vi "Run.vi"(8 "error in (no error)":errorcluster, 11 "Channel Rep in":refnum<class "Channel Rep.lvclass">) -> (0 "error out":errorcluster, 3 "Channel Rep out":refnum<class "Channel Rep.lvclass">)   [LabVIEW 2018, in "Channel Rep.lvclass"]
uses:
  Channel Rep.lvclass
  State Machine/State Machine.lvclass
  Socket2/Socket2/Socket2.lvclass
  RxTx/RxTx.lvclass
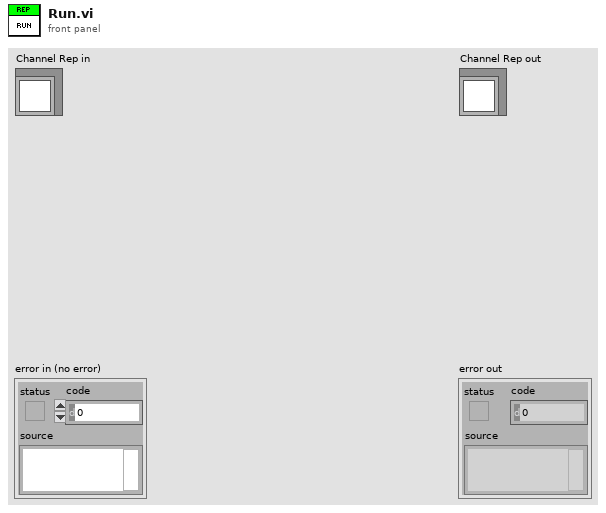
[diagram p1: front panel]
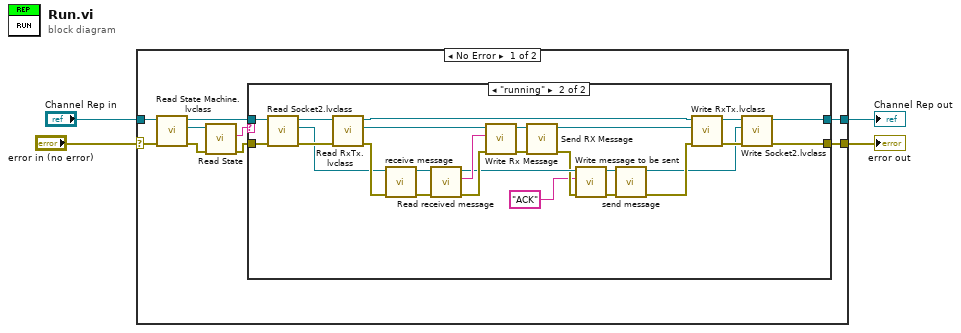
[diagram p0: block diagram]
diagram:
  n1 = case shown="No Error" "error in (no error)" {
    selector: "error in (no error)" -> [w12 w42]
    tunnel: "Channel Rep in" -> [w13 w43]
    tunnel: [w6 w43] -> w2
    tunnel: [w7 w42] -> w1
    frame No Error {
      n2 = call-dynamic "Read State Machine.lvclass.vi"("error in (no error)"=w12, "Communication Channel in"=w13) -> ("error out"=w11:errorcluster, "State Machine.lvclass"=w8:refnum<class "State Machine.lvclass">, "Communication Channel out"=w9:refnum<class "Channel Rep.lvclass">)  [unwired: 7 in]
      n3 = call-dynamic "Read State.vi"("error in (no error)"=w11, "State Machine in"=w8) -> ("error out"=w5:errorcluster, "State"=w10:string)  [unwired: 7 in, 1 out]
      n4 = case shown="\"running\"" w10 {
        tunnel: w9 -> [w15 w41]
        tunnel: [w15 w37] -> w6
        tunnel: [w14 w35] -> w7
        tunnel: w5 -> [w14 w34]
        frame Default {
        }
        frame "running" {
          n5 = call-dynamic "Read Socket2.lvclass.vi"("error in (no error)"=w34, "Communication Channel in"=w41) -> ("error out"=w39:errorcluster, "Socket2.lvclass"=w21:refnum<class "Socket2.lvclass">, "Communication Channel out"=w40:refnum<class "Channel Rep.lvclass">)  [unwired: 7 in]
          n6 = call-dynamic "Read RxTx.lvclass.vi"("error in (no error)"=w39, "Communication Channel in"=w40) -> ("error out"=w22:errorcluster, "RxTx.lvclass"=w23:refnum<class "RxTx.lvclass">, "Communication Channel out"=w33:refnum<class "Channel Rep.lvclass">)  [unwired: 7 in]
          n7 = call-dynamic "receive message.vi"("error in (no error)"=w22, "Socket in"=w21) -> ("error out"=w31:errorcluster, "Socket out"=w32:refnum<class "Socket2.lvclass">)  [unwired: 8 in]
          n8 = call-dynamic "Read received message.vi"("error in (no error)"=w31, "Socket in"=w32) -> ("error out"=w29:errorcluster, "received message"=w30:string, "Socket out"=w26:refnum<class "Socket2.lvclass">)  [unwired: 7 in]
          n9 = call "Write Rx Message.vi"("error in (no error)"=w29, "Rx Message"=w30, "RxTx in"=w23) -> ("error out"=w28:errorcluster, "RxTx out"=w27:refnum<class "RxTx.lvclass">)  [unwired: 7 in]
          n10 = call "Send RX Message.vi"("error in (no error)"=w28, "RxTx in"=w27) -> ("error out"=w18:errorcluster, "RxTx out"=w20:refnum<class "RxTx.lvclass">)  [unwired: 8 in]
          n11 = call-dynamic "Write message to be sent.vi"("error in (no error)"=w18, "message to be sent"="ACK", "Socket in"=w26) -> ("error out"=w24:errorcluster, "Socket out"=w25:refnum<class "Socket2.lvclass">)  [unwired: 7 in]
          n12 = call "send message.vi"("error in (no error)"=w24, "Socket in"=w25) -> ("error out"=w19:errorcluster, "Socket out"=w17:refnum<class "Socket2.lvclass">)  [unwired: 8 in]
          n13 = call-dynamic "Write RxTx.lvclass.vi"("error in (no error)"=w19, "RxTx.lvclass"=w20, "Communication Channel in"=w33) -> ("error out"=w36:errorcluster, "Communication Channel out"=w38:refnum<class "Channel Rep.lvclass">)  [unwired: 7 in]
          n14 = call-dynamic "Write Socket2.lvclass.vi"("error in (no error)"=w36, "Socket2.lvclass"=w17, "Communication Channel in"=w38) -> ("error out"=w35:errorcluster, "Communication Channel out"=w37:refnum<class "Channel Rep.lvclass">)  [unwired: 7 in]
        }
      }
    }
    frame Error {
    }
  }
  "Channel Rep out" <- w2
  "error out" <- w1
